vi "Get Request Type.vi"(8 "error in (no error)":errorcluster, 11 "GetProfileList in":refnum<class "GetProfileList.lvclass">) -> (0 "error out":errorcluster, 2 "Request Type":string, 3 "GetProfileList out":refnum<class "GetProfileList.lvclass">)   [LabVIEW 2020, in "obs-websocket.lvlib" / "GetProfileList.lvclass"]
uses:
  GetProfileList.lvclass
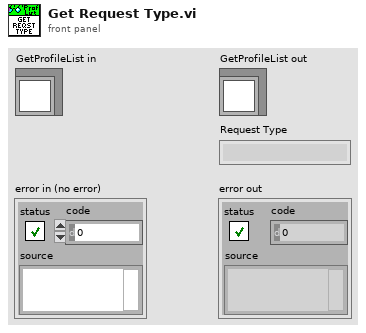
[diagram p1: front panel]
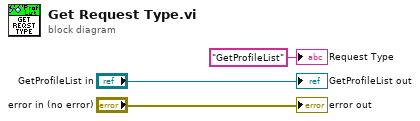
[diagram p0: block diagram]
diagram:
  "error out" <- "error in (no error)"
  "GetProfileList out" <- "GetProfileList in"
  "Request Type" <- "GetProfileList" ("Request Type")
